vi "Read Energy.vi"(8 "error in (no error)":errorcluster, 11 "Analyze Results Energy in":refnum<class "Analyze Results Energy.lvclass">) -> (0 "error out":errorcluster, 2 "Energy":dbl[unit], 3 "Analyze Results Energy out":refnum<class "Analyze Results Energy.lvclass">)   [LabVIEW 2014, in "Analyze Results Energy.lvclass"]
uses:
  Analyze Results Energy.lvclass
  Analyze Results Energy.lvclass/Analyze Results Energy.ctl
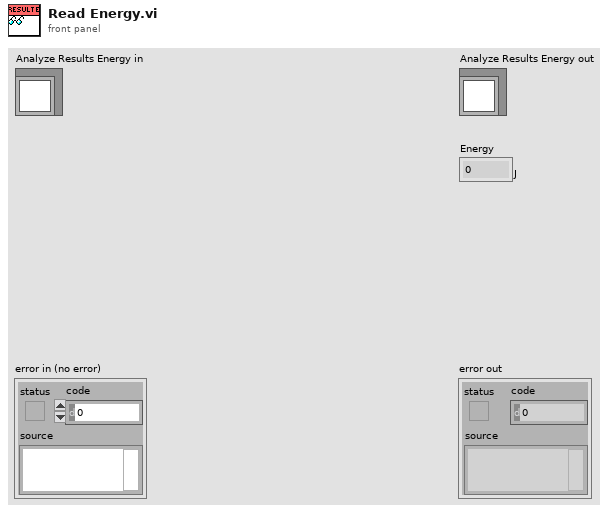
[diagram p1: front panel]
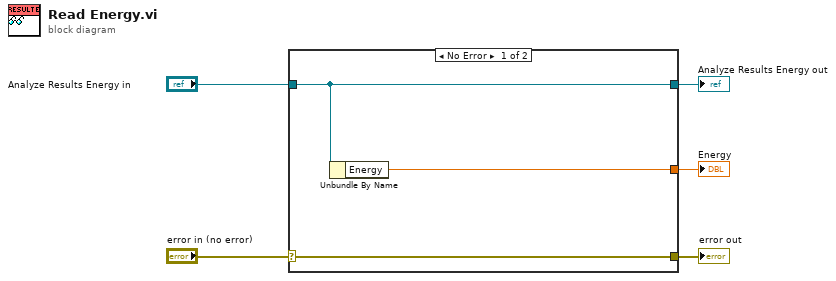
[diagram p0: block diagram]
diagram:
  n1 = case shown="No Error" "error in (no error)" {
    selector: "error in (no error)" -> [w8 w9]
    tunnel: [w8 w9] -> w4
    tunnel: [w7 w10] -> w2
    tunnel: "Analyze Results Energy in" -> [w7 w10]
    tunnel: [w6 _] -> w1
    frame No Error {
      n2 = Unbundle By Name(w7) -> ("Energy"=w6:dbl[unit])
    }
    frame Error {
    }
  }
  "error out" <- w4
  "Analyze Results Energy out" <- w2
  "Energy" <- w1
